vi "confPistofono.vi"(8 "error in (no error)":errorcluster) -> (0 "error out":errorcluster, 2 "PIST ref":refnum<visa-resource-name>, 3 "Pistofono out":refnum<class "Pistofono.lvclass">)   [LabVIEW 2019, in "Pistofono.lvclass"]
uses:
  Pistofono.lvclass
  Pistofono.lvclass/Pistofono.ctl
  <vilib>/Instr/_visa.llb/VISA Configure Serial Port (Instr).vi
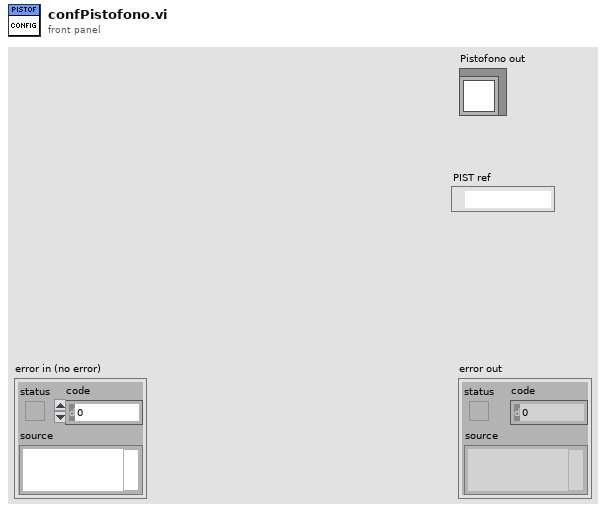
[diagram p1: front panel]
types:
  T1 = cluster{"baud rate":u32, "data bits":u16, "parity":enum16{"None", "Odd", "Even", "Mark", "Space"}, "stop bits":u16, "flow control":u16}
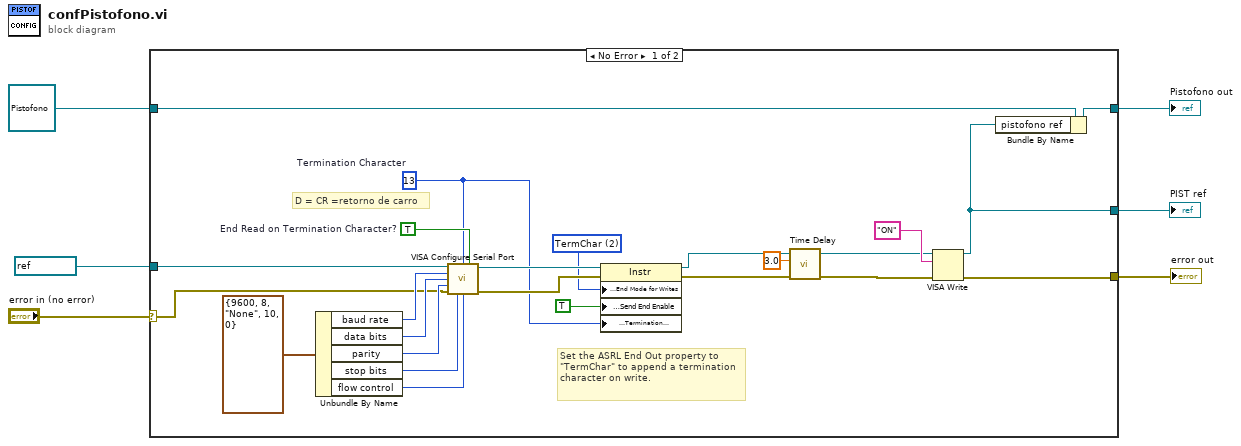
[diagram p0: block diagram]
diagram:
  n1 = case shown="No Error" "error in (no error)" {
    selector: "error in (no error)" -> [w15 w31]
    tunnel: [w11 w31] -> w5
    tunnel: [w16 w30] -> w3
    tunnel: refnum<class "Pistofono.lvclass"> refnum ("Pistofono in") -> [w29 w30]
    tunnel: [w10 _] -> w2
    tunnel: refnum<visa-resource-name> "COM3" ("VISA resource name") -> [w9 _]
    frame No Error {
      w19 = u8 13  # Termination Character
      w18 = u16 2 items=["None", "LastBit", "TermChar", "Break"] ("Serial Settings:Serial End Mode for Writes")
      w21 = TRUE  # End Read on Termination Character?
      # "D = CR =retorno de carro"
      # "Set the ASRL End Out property to \"TermChar\" to append a termination character on write."
      n2 = Unbundle By Name(T1 {"baud rate"=9600, "data bits"=8, "parity"=enum."None", "stop bits"=10, "flow control"=0} ("Serial Settings")) -> ("baud rate"=w23:u32, "data bits"=w24:u16, "parity"=w25:enum16{"None", "Odd", "Even", "Mark", "Space"}, "stop bits"=w26:u16, "flow control"=w20:u16)
      n3 = call-poly "VISA Configure Serial Port"("VISA resource name"=w9, "termination char\n(0xA = '\\n' = LF)"=w19, "Enable Termination\nChar (T)"=w21, "baud rate (9600)"=w23, "data bits (8)"=w24, "parity (0:none)"=w25, "error in (no error)"=w15, "stop bits (10: 1 bit)"=w26, "flow control (0:none)"=w20) -> ("VISA resource name out"=w27:refnum<visa-resource-name>, "error out"=w28:errorcluster)  [unwired: 1 in, 4 out]
      n4 = property class="Instr"(reference=w27, error in=w28, "Serial Settings:End Mode for Writes"=w18, "Message Based Settings:Send End Enable"=TRUE, "Message Based Settings:Termination Character"=w19) -> (reference out=w12:refnum<visa-resource-name>, error out=w13:errorcluster)
      n5 = call "Time Delay"("error in (no error)"=w13, "Delay Time (s)"=3.0) -> ("error out"=w8:errorcluster)  [unwired: 9 in]
      n6 = VISA Write(VISA resource name=w12, write buffer="ON" ("Command"), error in (no error)=w8) -> (VISA resource name out=w10:refnum<visa-resource-name>, error out=w11:errorcluster)  [unwired: 1 out]
      n7 = Bundle By Name(cluster=w29, "pistofono ref"=w10) -> (w16:refnum<class "Pistofono.lvclass">)
    }
    frame Error {
    }
  }
  "error out" <- w5
  "Pistofono out" <- w3
  "PIST ref" <- w2
